vi "ReadPlugins.vi"(1 "Section":string, 2 "MenuName":string="Plugins", 3 "Menu Refnum":refnum<k9>) -> ()   [LabVIEW 2014]
doc: "Use this template to build a standard state machine design pattern. Each state executes code and determines which state to transition to. Contrast this design pattern with the user interface event pattern, in which code executes in response to user actions. Contrast this design pattern also with the queued message handler pattern, in which each message handling code can queue zero or more new messages."
uses:
  globals/AzCamGlobals.vi
  <vilib>/Utility/config.llb/Read Key (String).vi
  <vilib>/Utility/config.llb/NI_LVConfig.lvlib
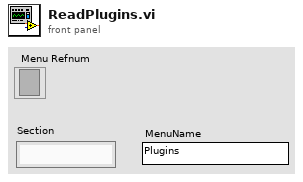
[diagram p1: front panel]
types:
  T1 = typedef "NI_LVConfig.lvlib/Config Data RefNum.ctl" = refnum<k1>
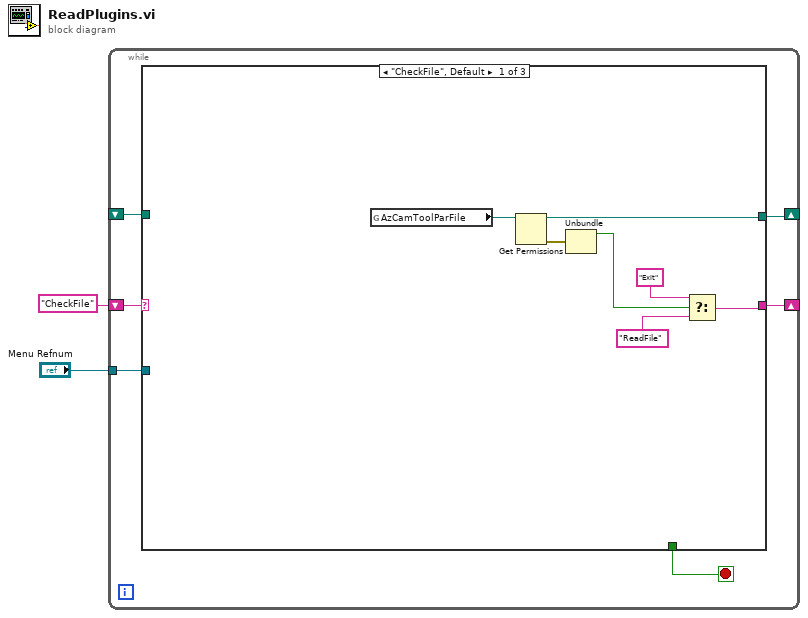
[diagram p0: block diagram]
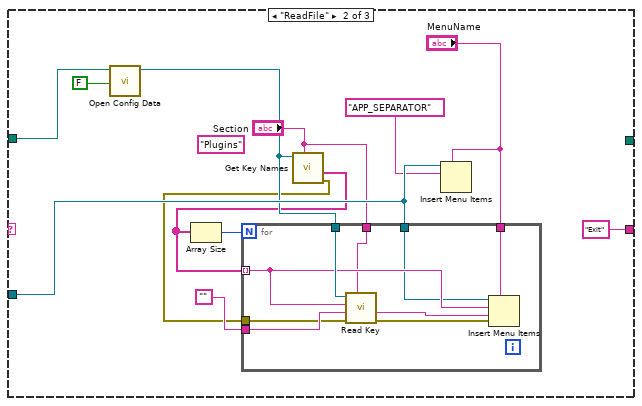
[diagram p2: hidden frame]
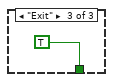
[diagram p3: hidden frame]
diagram:
  n1 = while {
    shift-right: [w6] -> _
    shift-left: "CheckFile" -> [w7]
    tunnel: "Menu Refnum" -> [w5]
    shift-right: [w4] -> _
    shift-left: _ -> [w3]
    stop <- w8 stop-if-true
    n2 = case shown="\"CheckFile\", Default" w7 {
      tunnel: [_ _ TRUE] -> w8
      tunnel: [w11 "Exit" _] -> w6
      tunnel: w5 -> [_ w24 _]
      tunnel: [w10 _ _] -> w4
      tunnel: w3 -> [_ w25 _]
      frame "CheckFile", Default {
        n3 = global read "AzCamGlobals.vi" "AzCamToolParFile"() -> (w9:path)
        n4 = Get Permissions(11:w9) -> (0:w15:errorcluster, 3:w10:path)  [unwired: 1 in, 3 out]
        n5 = Unbundle(w15) -> ("status"=w14:bool)  [unwired: 2 out]
        n6 = Select(t="Exit", s=w14, f="ReadFile") -> (s? t:f=w11:string)
      }
      frame "ReadFile" {
        (unwired) "Plugins" ("String")
        n7 = call <vilib>:"Open Config Data.vi"("create file if necessary (T)"=FALSE ("create file if necessary? (T)"), "configuration file path"=w25) -> ("refnum"=w21:T1)  [unwired: 7 in, 2 out]
        n8 = call <vilib>:"Get Key Names.vi"("section"="Section", "refnum"=w21) -> ("error out"=w18:errorcluster, "key names"=w17:string[])  [unwired: 6 in, 2 out]
        n9 = Array Size(array=w17) -> (size(s)=w20:i32)
        n10 = for {
          N: w20 -> [_]
          tunnel: w17 -> [w33] mode=indexing
          tunnel: "" -> [w36]
          tunnel: w21 -> [w35]
          tunnel: "Section" -> [w30]
          tunnel: w18 -> [w31]
          tunnel: "MenuName" -> [w29]
          tunnel: w24 -> [w28]
          n11 = call-poly <vilib>:"Read Key.vi"("section"=w30, "error in (no error)"=w31, "default value"=w36, "key"=w33, "refnum"=w35) -> ("error out"=w32:errorcluster, "value"=w34:string)  [unwired: 3 in, 2 out]
          n12 = Insert Menu Items(5:w29, 6:w32, 7:w34, 8:w33, 9:w28) -> ()  [unwired: 1 in, 3 out]
        }
        n13 = Insert Menu Items(5:"MenuName", 8:"APP_SEPARATOR", 9:w24) -> ()  [unwired: 3 in, 3 out]
      }
      frame "Exit" {
      }
    }
  }
